vi "0_9 NUMBER TO STRING(SubVI).vi"(1 "A":i32) -> (0 "element":string)   [LabVIEW 2019]
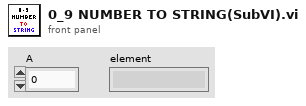
[diagram p1: front panel]
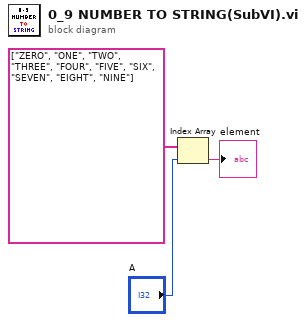
[diagram p0: block diagram]
diagram:
  n1 = Index Array(array=string[] ["ZERO", "ONE", "TWO", "THREE", "FOUR", "FIVE", "SIX", "SEVEN", "EIGHT", "NINE"], index="A") -> (element=→"element":string)
